vi "Write Attributes Metadata in Actor.vi"(7 "Actor in":refnum<class "Actor.lvclass">, 10 "Attributes Metadata":refnum<class "Attributes Metadata.lvclass">) -> (5 "Actor out":refnum<class "Actor.lvclass">)   [LabVIEW 2020, in "jettl.lvlib"]
uses:
  jettl.lvlib
  Actor/Actor.lvclass
  Attributes Metadata/Attributes Metadata.lvclass
  Attributes/Attributes.lvclass
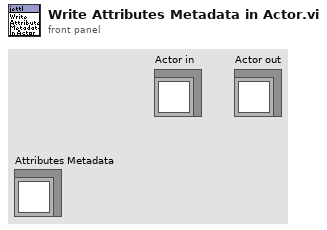
[diagram p1: front panel]
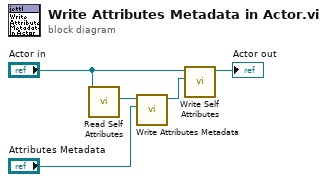
[diagram p0: block diagram]
diagram:
  n1 = call-dynamic "Read Self Attributes.vi"("Actor in"="Actor in") -> ("Self Attributes"=w3:refnum<class "Attributes.lvclass">)  [unwired: 10 in]
  n2 = call-dynamic "Write Attributes Metadata.vi"("Attributes Metadata"="Attributes Metadata", "Attributes in"=w3) -> ("Attributes out"=w2:refnum<class "Attributes.lvclass">)  [unwired: 9 in]
  n3 = call-dynamic "Write Self Attributes.vi"("Self Attributes"=w2, "Actor in"="Actor in") -> ("Actor out"=→"Actor out":refnum<class "Actor.lvclass">)  [unwired: 9 in]
